vi "Populate XYGraphs.vi"(8 "error in (no error)":errorcluster, 9 "Array":dbl[][](array[numeric]), 10 "Red":refnum<vi>, 11 "Blue":refnum<vi>) -> (0 "error out":errorcluster)   [LabVIEW 2013, in "main.lvlib"]
uses:
  main.lvlib
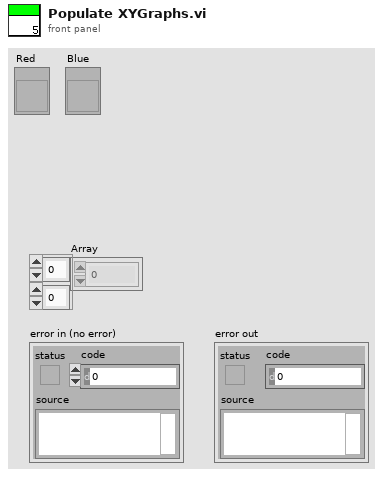
[diagram p1: front panel]
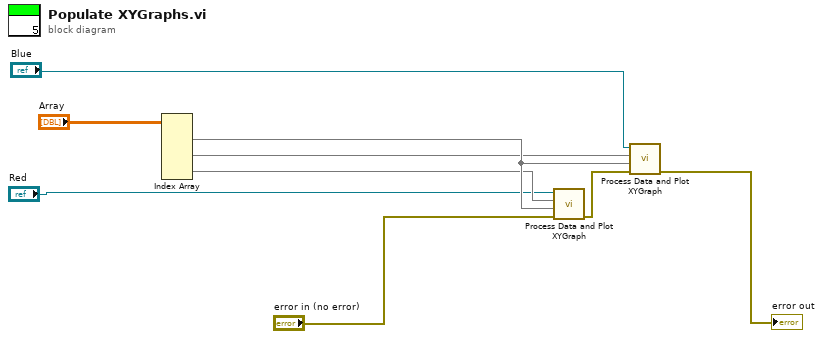
[diagram p0: block diagram]
diagram:
  n1 = Index Array(array="Array") -> (element #1=w5:dbl[], element #2=w3:dbl[], element #3=w4:dbl[])  [unwired: 6 in]
  n2 = call "Process Data and Plot XYGraph.vi"("error in (no error)"="error in (no error)", "Pressure"=w5, "Graph"=w4, "WaveformGraph in"="Red") -> ("error out"=w8:errorcluster)  [unwired: 7 in]
  n3 = call "Process Data and Plot XYGraph.vi"("error in (no error)"=w8, "Pressure"=w5, "Graph"=w3, "WaveformGraph in"="Blue") -> ("error out"=→"error out":errorcluster)  [unwired: 7 in]
